vi "Wait For LACK OF Front Panel Activity.vi"(1 "Delay (ms)":u32=1000, 2 "Ctl Refnum":refnum<vi>) -> ()   [LabVIEW 2013]
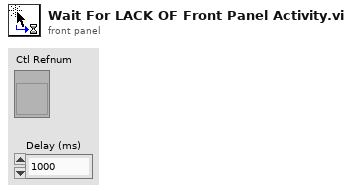
[diagram p1: front panel]
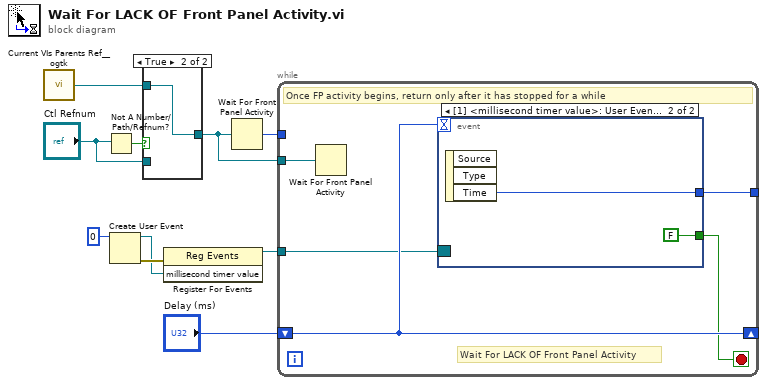
[diagram p0: block diagram]
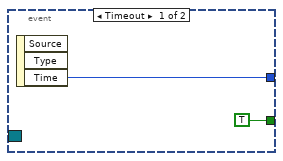
[diagram p3: hidden frame]
diagram:
  n1 = call <userlib>:"Current VIs Parents Ref__ogtk.vi"() -> ("Calling VI's Reference"=w3:refnum<vi>)  [unwired: 2 in]
  n2 = Not A Number/Path/Refnum?(number/path/refnum="Ctl Refnum") -> (NaN/Path/Refnum?=w4:bool)
  n3 = Create User Event(user event datatype=u32 0 ("millisecond timer value")) -> (user event=w6:refnum<user-event>, error out=w7:errorcluster)  [unwired: 1 in]
  n4 = case shown="True" w4 {
    tunnel: w3 -> [_ w12]
    tunnel: "Ctl Refnum" -> [w11 _]
    tunnel: [w11 w12] -> w1
    frame False {
    }
    frame True {
    }
  }
  n5 = register-events(error in=w7, w6) -> (reference out=w8:refnum<event-registration>)  [unwired: 1 in, 1 out]
  n6 = Wait For Front Panel Activity(2:w1) -> (0:w10:u32)  [unwired: 2 in]
  n7 = while {
    tunnel: w10 -> [_]
    shift-right: [w17] -> _
    shift-left: "Delay (ms)" -> [w17]
    tunnel: w1 -> [w13]
    tunnel: [w15] -> _
    tunnel: w8 -> [w14]
    stop <- w16 stop-if-true
    # "Wait For LACK OF Front Panel Activity"
    # "Once FP activity begins, return only after it has stopped for a while"
    n8 = Wait For Front Panel Activity(2:w13) -> ()  [unwired: 2 in, 1 out]
    n9 = event shown="[1] <millisecond timer value>: User Event" {
      selector: w14 -> [_ _]
      dyn-events: _ -> [_ _]
      timeout: w17 -> [_ _]
      tunnel: [TRUE FALSE] -> w16
      tunnel: [w18 w20] -> w15
      event Timeout {
        n10 = event-data() -> ("Time"=w18:u32)  [unwired: 1 in, 2 out]
      }
      event User Event {
        n11 = event-data() -> ("Time"=w20:u32)  [unwired: 1 in, 2 out]
      }
    }
  }
